vi "Target Send to Logging v2.vi"(8 "Valid for Logging or Not?":bool, 9 "rt fifo":refnum<k33>, 10 "Target Lossy Data":T1) -> ()   [LabVIEW 2018]
uses:
  Target Lossy Data.ctl
  Sensor Data.ctl
  Target Logging Cluster.ctl
  Logging Data Cluster.ctl
  Target Logging Control Signals.ctl
  Target Logging Sensors.ctl
panel:
  out "error out":errorcluster
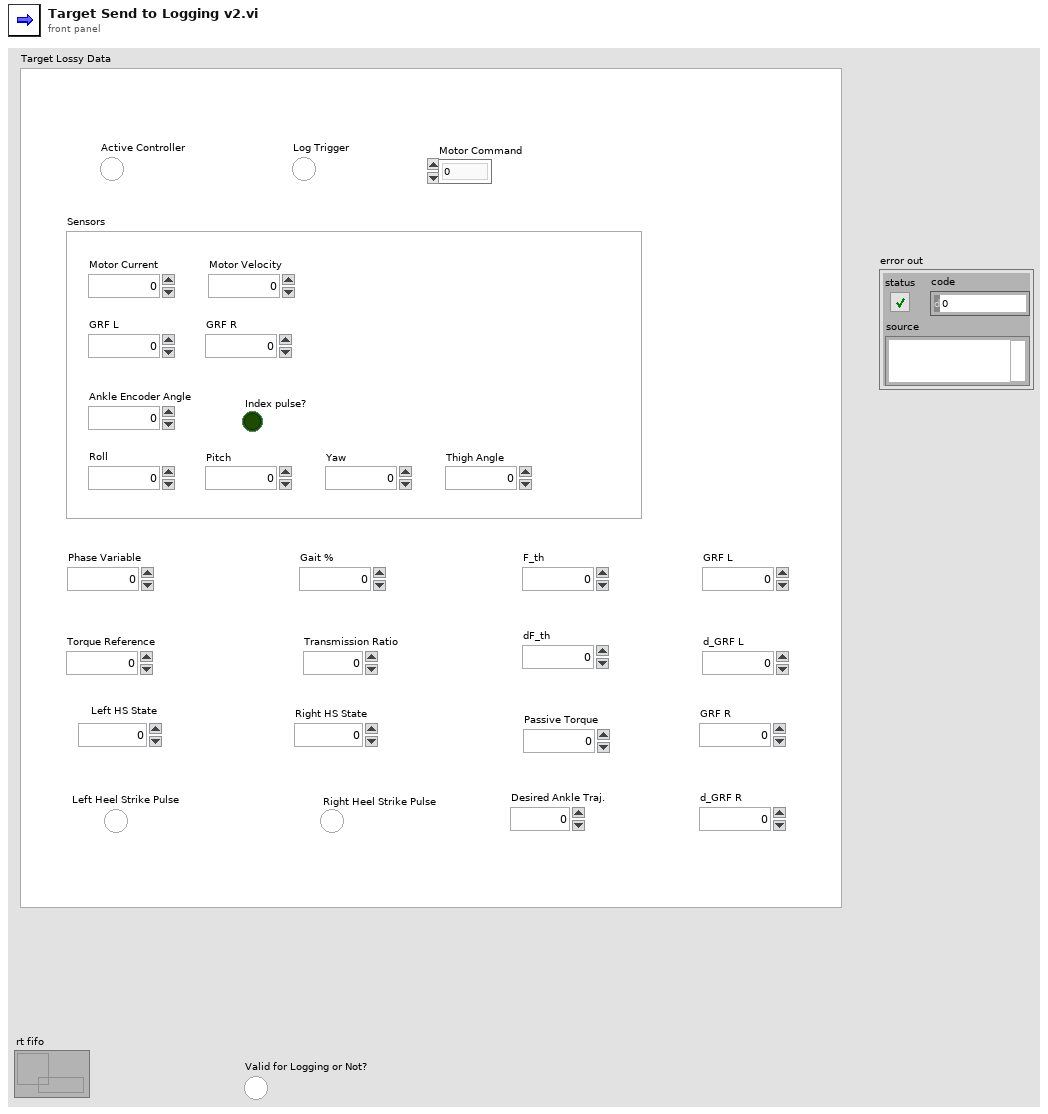
[diagram p1: front panel]
types:
  T1 = typedef "Target Lossy Data.ctl" = cluster{"Active Controller":bool, "Log Trigger":bool, "Sensors":T2, "Motor Command":dbl, "Phase Variable":dbl, "Left HS State":u32, "Left Heel Strike Pulse":bool, "Gait %":dbl, "Torque Reference":dbl, "Passive Torque":dbl, "F_th":dbl, "dF_th":dbl, "d_GRF L":dbl, "GRF L":dbl, "Transmission Ratio":dbl, "Desired Ankle Traj.":dbl, "Right HS State":u32, "Right Heel Strike Pulse":bool, "d_GRF R":dbl, "GRF R":dbl}
  T2 = typedef "Sensor Data.ctl" = cluster{"Motor Current":dbl, "Motor Velocity":dbl, "Ankle Encoder Angle":dbl, "GRF L":dbl, "GRF R":dbl, "Index pulse?":bool, "Roll":dbl, "Pitch":dbl, "Yaw":dbl, "Thigh Angle":dbl}
  T3 = typedef "Logging Data Cluster.ctl" = cluster{"Control Signals":T4, "Target Sensors":T5}
  T4 = typedef "Target Logging Control Signals.ctl" = cluster{"Phi":dbl, "Gait %":dbl, "ILC Desired Ankle Angle":dbl, "Desired Motor Current":dbl, "Transmission Ratio":dbl, "Passive Torque Estimate":dbl, "Torque Reference":dbl, "Left HS?":bool, "Left HS State":u32, "Right HS?":bool, "Right HS State":u32, "dGRF L":dbl, "dGRF R":dbl, "GRF L (filt) ":dbl, "GRF R (filt)":dbl}
  T5 = typedef "Target Logging Sensors.ctl" = cluster{"Sensors":T2}
  T6 = typedef "Target Logging Cluster.ctl" = cluster{"Valid for Logging?":bool, "Data":T3}
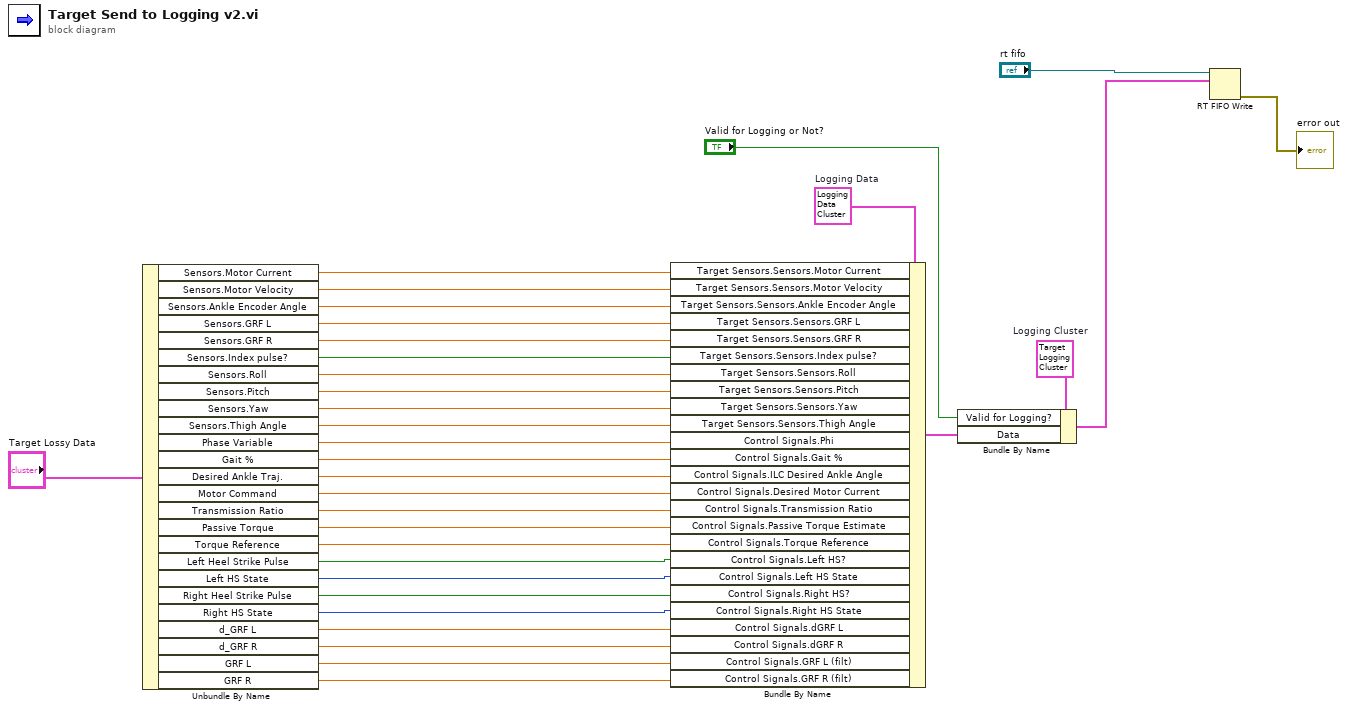
[diagram p0: block diagram]
diagram:
  w29 = T3 {"Control Signals"={"Phi"=0.0, "Gait %"=0.0, "ILC Desired Ankle Angle"=0.0, "Desired Motor Current"=0.0, "Transmission Ratio"=0.0, "Passive Torque Estimate"=0.0, "Torque Reference"=0.0, "Left HS?"=FALSE, "Left HS State"=0, "Right HS?"=FALSE, "Right HS State"=0, "dGRF L"=0.0, "dGRF R"=0.0, "GRF L (filt) "=0.0, "GRF R (filt)"=0.0}, "Target Sensors"={"Sensors"={"Motor Current"=0.0, "Motor Velocity"=0.0, "Ankle Encoder Angle"=0.0, "GRF L"=0.0, "GRF R"=0.0, "Index pulse?"=FALSE, "Roll"=0.0, "Pitch"=0.0, "Yaw"=0.0, "Thigh Angle"=0.0}}}  # Logging Data
  w31 = T6 {"Valid for Logging?"=FALSE, "Data"={"Control Signals"={"Phi"=0.0, "Gait %"=0.0, "ILC Desired Ankle Angle"=0.0, "Desired Motor Current"=0.0, "Transmission Ratio"=0.0, "Passive Torque Estimate"=0.0, "Torque Reference"=0.0, "Left HS?"=FALSE, "Left HS State"=0, "Right HS?"=FALSE, "Right HS State"=0, "dGRF L"=0.0, "dGRF R"=0.0, "GRF L (filt) "=0.0, "GRF R (filt)"=0.0}, "Target Sensors"={"Sensors"={"Motor Current"=0.0, "Motor Velocity"=0.0, "Ankle Encoder Angle"=0.0, "GRF L"=0.0, "GRF R"=0.0, "Index pulse?"=FALSE, "Roll"=0.0, "Pitch"=0.0, "Yaw"=0.0, "Thigh Angle"=0.0}}}}  # Logging Cluster
  n1 = Unbundle By Name("Target Lossy Data") -> ("Sensors.Motor Current"=w9:dbl, "Sensors.Motor Velocity"=w10:dbl, "Sensors.Ankle Encoder Angle"=w11:dbl, "Sensors.GRF L"=w12:dbl, "Sensors.GRF R"=w13:dbl, "Sensors.Index pulse?"=w14:bool, "Sensors.Roll"=w15:dbl, "Sensors.Pitch"=w16:dbl, "Sensors.Yaw"=w17:dbl, "Sensors.Thigh Angle"=w18:dbl, "Phase Variable"=w26:dbl, "Gait %"=w25:dbl, "Desired Ankle Traj."=w24:dbl, "Motor Command"=w23:dbl, "Transmission Ratio"=w22:dbl, "Passive Torque"=w21:dbl, "Torque Reference"=w20:dbl, "Left Heel Strike Pulse"=w8:bool, "Left HS State"=w7:u32, "Right Heel Strike Pulse"=w6:bool, "Right HS State"=w5:u32, "d_GRF L"=w4:dbl, "d_GRF R"=w3:dbl, "GRF L"=w2:dbl, "GRF R"=w1:dbl)
  n2 = Bundle By Name(cluster=w29, "Target Sensors.Sensors.Motor Current"=w9, "Target Sensors.Sensors.Motor Velocity"=w10, "Target Sensors.Sensors.Ankle Encoder Angle"=w11, "Target Sensors.Sensors.GRF L"=w12, "Target Sensors.Sensors.GRF R"=w13, "Target Sensors.Sensors.Index pulse?"=w14, "Target Sensors.Sensors.Roll"=w15, "Target Sensors.Sensors.Pitch"=w16, "Target Sensors.Sensors.Yaw"=w17, "Target Sensors.Sensors.Thigh Angle"=w18, "Control Signals.Phi"=w26, "Control Signals.Gait %"=w25, "Control Signals.ILC Desired Ankle Angle"=w24, "Control Signals.Desired Motor Current"=w23, "Control Signals.Transmission Ratio"=w22, "Control Signals.Passive Torque Estimate"=w21, "Control Signals.Torque Reference"=w20, "Control Signals.Left HS?"=w8, "Control Signals.Left HS State"=w7, "Control Signals.Right HS?"=w6, "Control Signals.Right HS State"=w5, "Control Signals.dGRF L"=w4, "Control Signals.dGRF R"=w3, "Control Signals.GRF L (filt)"=w2, "Control Signals.GRF R (filt)"=w1) -> (w28:T3)
  n3 = Bundle By Name(cluster=w31, "Valid for Logging?"="Valid for Logging or Not?", "Data"=w28) -> (w30:T6)
  n4 = RT FIFO Write(0:"rt fifo", 1:w30) -> (11:→"error out":errorcluster)  [unwired: 3 in, 3 out]
